vi "fast_fourier_transform.vi"() -> ()   [LabVIEW 2020]
uses:
  <vilib>/Analysis/2dsp.llb/Real FFT.vi
  <vilib>/Analysis/NI_AALPro.lvlib
panel:
  in  "shift?":bool
  in  "FFT size":i32=-1
  out "Fast Fourier Transform Graph":dbl[](graph)
  out "Amplitude vs Time (Chart)":waveform(dbl)(graph)
  out "Amplitude vs Time (Graph)":waveform(dbl)(graph)
  in  "path":path
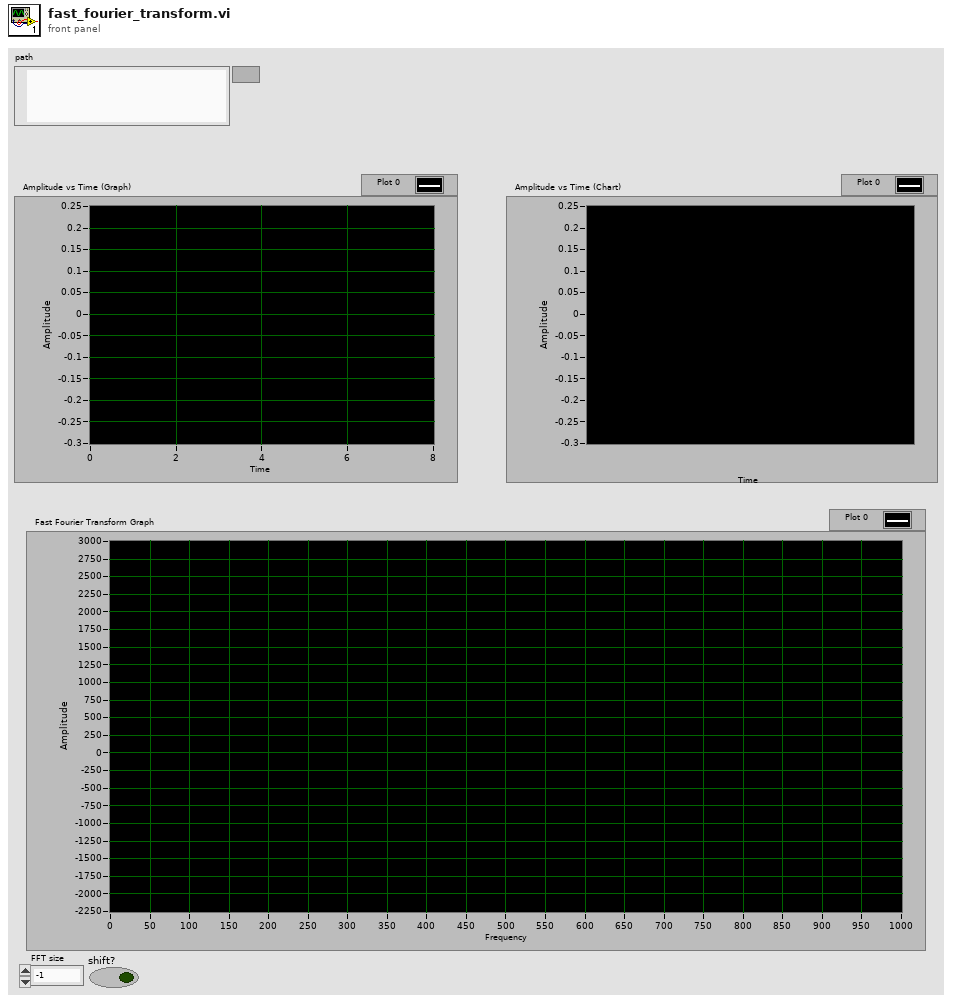
[diagram p1: front panel]
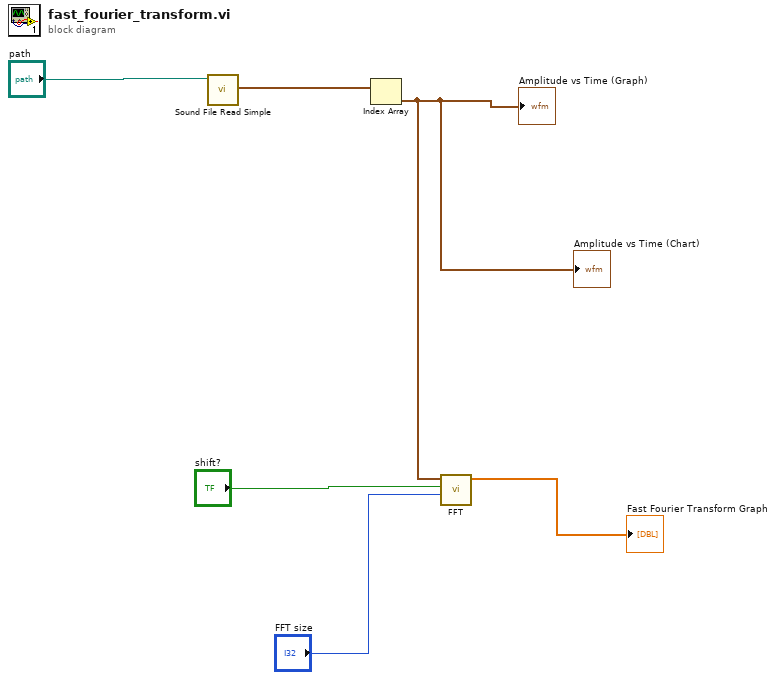
[diagram p0: block diagram]
diagram:
  n1 = call <vilib>:"Sound File Read Simple.vi"("path"="path") -> ("data"=w5:waveform(dbl)[])  [unwired: 7 in, 3 out]
  n2 = Index Array(array=w5) -> (element=w4:waveform(dbl))  [unwired: 1 in]
  "Amplitude vs Time (Graph)" <- w4
  "Amplitude vs Time (Chart)" <- w4
  n3 = call-poly <vilib>:"FFT.vi"("FFT size"="FFT size", "shift?"="shift?", "X"=w4) -> ("FFT {X}"=→"Fast Fourier Transform Graph":cdb[])  [unwired: 7 in, 1 out]
